vi "Prepare Control.vi"(7 "VolatusAPI":refnum<class "VolatusAPI.lvclass">, 8 "error in (no error)":errorcluster, 11 "ValveControl in":refnum<class "MultiControl.lvclass">) -> (0 "error out":errorcluster, 3 "ValveControl out":refnum<class "MultiControl.lvclass">)   [LabVIEW 2020, in "VolatusControl.lvlib" / "MultiControl.lvclass"]
uses:
  MultiControl.lvclass
  Volatus/VolatusAPI/VolatusAPI.lvclass
  MultiControl.lvclass/MultiControl.ctl
  <vilib>/Utility/miscctls.llb/LVMapReplaceAction.ctl
  Volatus/Module Identity/Module Identity.lvclass/Module Identity.ctl
  Volatus/Module Identity/Create.vi
  Volatus/Module Identity/Module Identity.lvclass
  C:/dev/lv20CE/relink/lv-volatus/Volatus/Identity/Identity.lvclass
  Volatus/VolatusAPI/Lookup Channel Info.vi
  Volatus/VolatusAPI/Lookup Q.vi
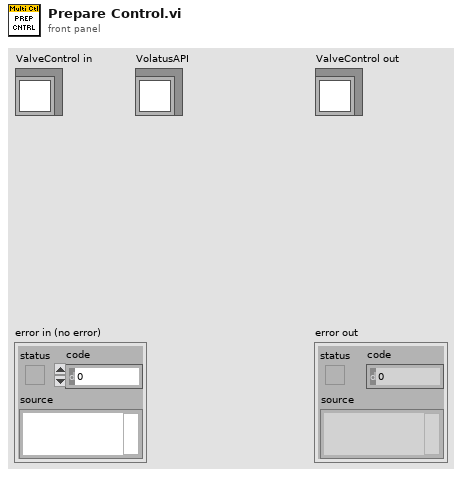
[diagram p1: front panel]
types:
  T1 = typedef "LVMapReplaceAction.ctl" = enum32{"Modify Entry only if found", "Add or Modify Entry", "Delete Entry"}
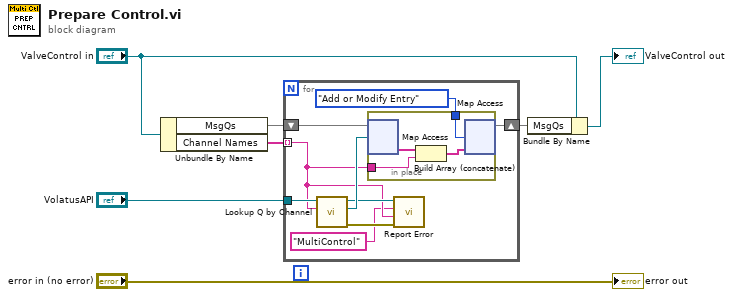
[diagram p0: block diagram]
diagram:
  n1 = Unbundle By Name("ValveControl in") -> ("MsgQs"=w5:map{refnum<class "MessageQ.lvclass">, string[]}, "Channel Names"=w4:string[])
  n2 = for {
    shift-right: [w9] -> w1
    shift-left: w5 -> [w15]
    tunnel: w4 -> [w11] mode=indexing
    tunnel: "VolatusAPI" -> [w16]
    n3 = call "Lookup Q by Channel.vi"("Channel Name"=w11, "VolatusAPI in"=w16) -> ("error out"=w12:errorcluster, "MessageQ"=w14:refnum<class "MessageQ.lvclass">, "VolatusAPI out"=w13:refnum<class "VolatusAPI.lvclass">)  [unwired: 7 in]
    n4 = in-place {
      in-place-border: w11 -> [w19]
      in-place-border: LVMapReplaceAction."Add or Modify Entry" ("action") -> [w17]
      n5 = in-place-map #1(w15, w14) -> (w20:string[])  [unwired: 1 in, 1 out]
      n6 = Build Array (concatenate)(w20, w19) -> (w18:string[])
      n7 = in-place-map #1(w18, w17) -> (w9:map{refnum<class "MessageQ.lvclass">, string[]})  [unwired: 2 out]
    }
    n8 = call "Report Error.vi"("error in (no error)"=w12, "Message"=w11, "Context"="MultiControl", "VolatusAPI in"=w13) -> ()  [unwired: 6 in, 2 out]
  }
  n9 = Bundle By Name(cluster="ValveControl in", "MsgQs"=w1) -> (→"ValveControl out":refnum<class "MultiControl.lvclass">)
  "error out" <- "error in (no error)"
